vi "FPGA_main.vi"() -> ()   [LabVIEW 2019]
uses:
  trigger.ctl
  state.ctl
  <vilib>/rvi/Emulation/niFpgaGetClockAttributes.vi
  <vilib>/rvi/Emulation/niFpgaSctlEmulationGetInTimedLoop.vi
  <vilib>/rvi/Emulation/niFpgaEmulationReportErrorSimple.vi
  <vilib>/rvi/eio/common/nirviEmuTemplateMethod_errors.vi
  <vilib>/rvi/Emulation/niFpgaEmulationIsFPGAContextNoSignature.vi
  <vilib>/rvi/DataTransferAndStorage/Container/Common/niFpgaContainerGetUniqueNameForEmu.vi
  <vilib>/rvi/Memory/Memory_Emulation/niFpgaMemoryEmulationCacheClearOnFirstRun.vi
  <vilib>/rvi/Memory/Memory_Emulation/nirvimemoryEmulationManagerCache_MakeExclusive.vi
  <vilib>/rvi/Memory/Memory_Emulation/niFpgaMemoryEmulationValidateCache.vi
  <vilib>/rvi/Memory/Memory_Emulation/nirvimemoryEmulationManagerCache_InsertValue.vi
  <vilib>/Utility/error.llb/Clear Errors.vi
  <vilib>/rvi/Memory/Memory_Emulation/nirvimemoryEmulationManagerCache_ReleaseExclusive.vi
  <vilib>/rvi/Memory/Memory_Emulation/nirvimemoryEmulationManagerCache_GetValue.vi
  <vilib>/rvi/Memory/Memory_Emulation/nirvimemoryEmulationManagerCache_SetValue.vi
  <vilib>/rvi/Emulation/niFpgaProcessEmulError.vi
  <vilib>/rvi/Memory/Memory_Emulation/nirvimemoryFastEmulation.vi
  <vilib>/rvi/Memory/Memory_Emulation/nirvimemoryEmulation.vi
  <vilib>/rvi/errors/nirviReportUnexpectedCaseInternalError (U32).vi
  <vilib>/rvi/errors/niFpgaSetErrorForExecOnDevCompSimple.vi
  <vilib>/rvi/eio/common/nirviEmuReportErrorAndStop.vi
  <vilib>/rvi/FIFO/Fifo_Resource/nirvififoEmulationSetSize.vi
  <vilib>/rvi/FIFO/Fifo_Resource/nirviFifoEmulationQueueMgr.vi
  <instcachedir>/0/nirviFifoEmulationQueueMgr_E5CAEC123FF24DC58D834DCA3CDAA9B5.lvgen/nirviFifoEmulationQueueMgr_E5CAEC123FF24DC58D834DCA3CDAA9B5_002.vi
  <vilib>/rvi/FIFO/Fifo_Resource/nirvififoEmulationDetermineInputValidOut.vi
  <vilib>/rvi/FIFO/Fifo_Resource/nirvififoEmulationCreateLock.vi
  <vilib>/rvi/FIFO/Fifo_Resource/nirvififoEmulationObtainLock.vi
  <vilib>/rvi/FIFO/Fifo_Resource/nirvififoEmulationReleaseLock.vi
  <vilib>/rvi/occurrence/nirviWaitOnOccurrenceBase.vi
  <vilib>/rvi/errors/nirviReportUnexpectedCaseInternalError.vi
  <vilib>/rvi/Emulation/niFpgaCriticalErrorInLSC.vi
  <vilib>/rvi/interface/RandomDataEmulation/niFpgaRandomDataHandleErrors.vi
  <vilib>/eio/EIONode/EIONode.xnode
  <vilib>/rvi/DataTransferAndStorage/Container/XNode/niFpgaContainer.xnode
  <vilib>/rvi/DataTransferAndStorage/Register/Emulation/niFpgaRegisterEmulation.vi
  <vilib>/rvi/FIFO/Fifo_Resource/nirvififoEmulationWrite.vi
  <vilib>/rvi/FIFO/Fifo_Resource/nirvififoEmulationRead.vi
  <vilib>/rvi/interface/RandomDataEmulation/nirviRandomDataFpgaReadWriteTemplate.vi
panel:
  out "Numeric":u32
  in  "Samples":i16
  in  "Trigger":T1
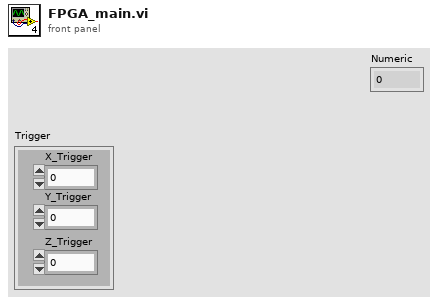
[diagram p1: front panel]
types:
  T1 = typedef "trigger.ctl" = cluster{"X_Trigger":i16, "Y_Trigger":i16, "Z_Trigger":i16}
  T2 = typedef "state.ctl" = enum16{"Send_fifo", "Send_memo", "Wait"}
  T3 = cluster{"X_Trigger":i16, "Y_Trigger":i16, "Z_Trigger":i16}
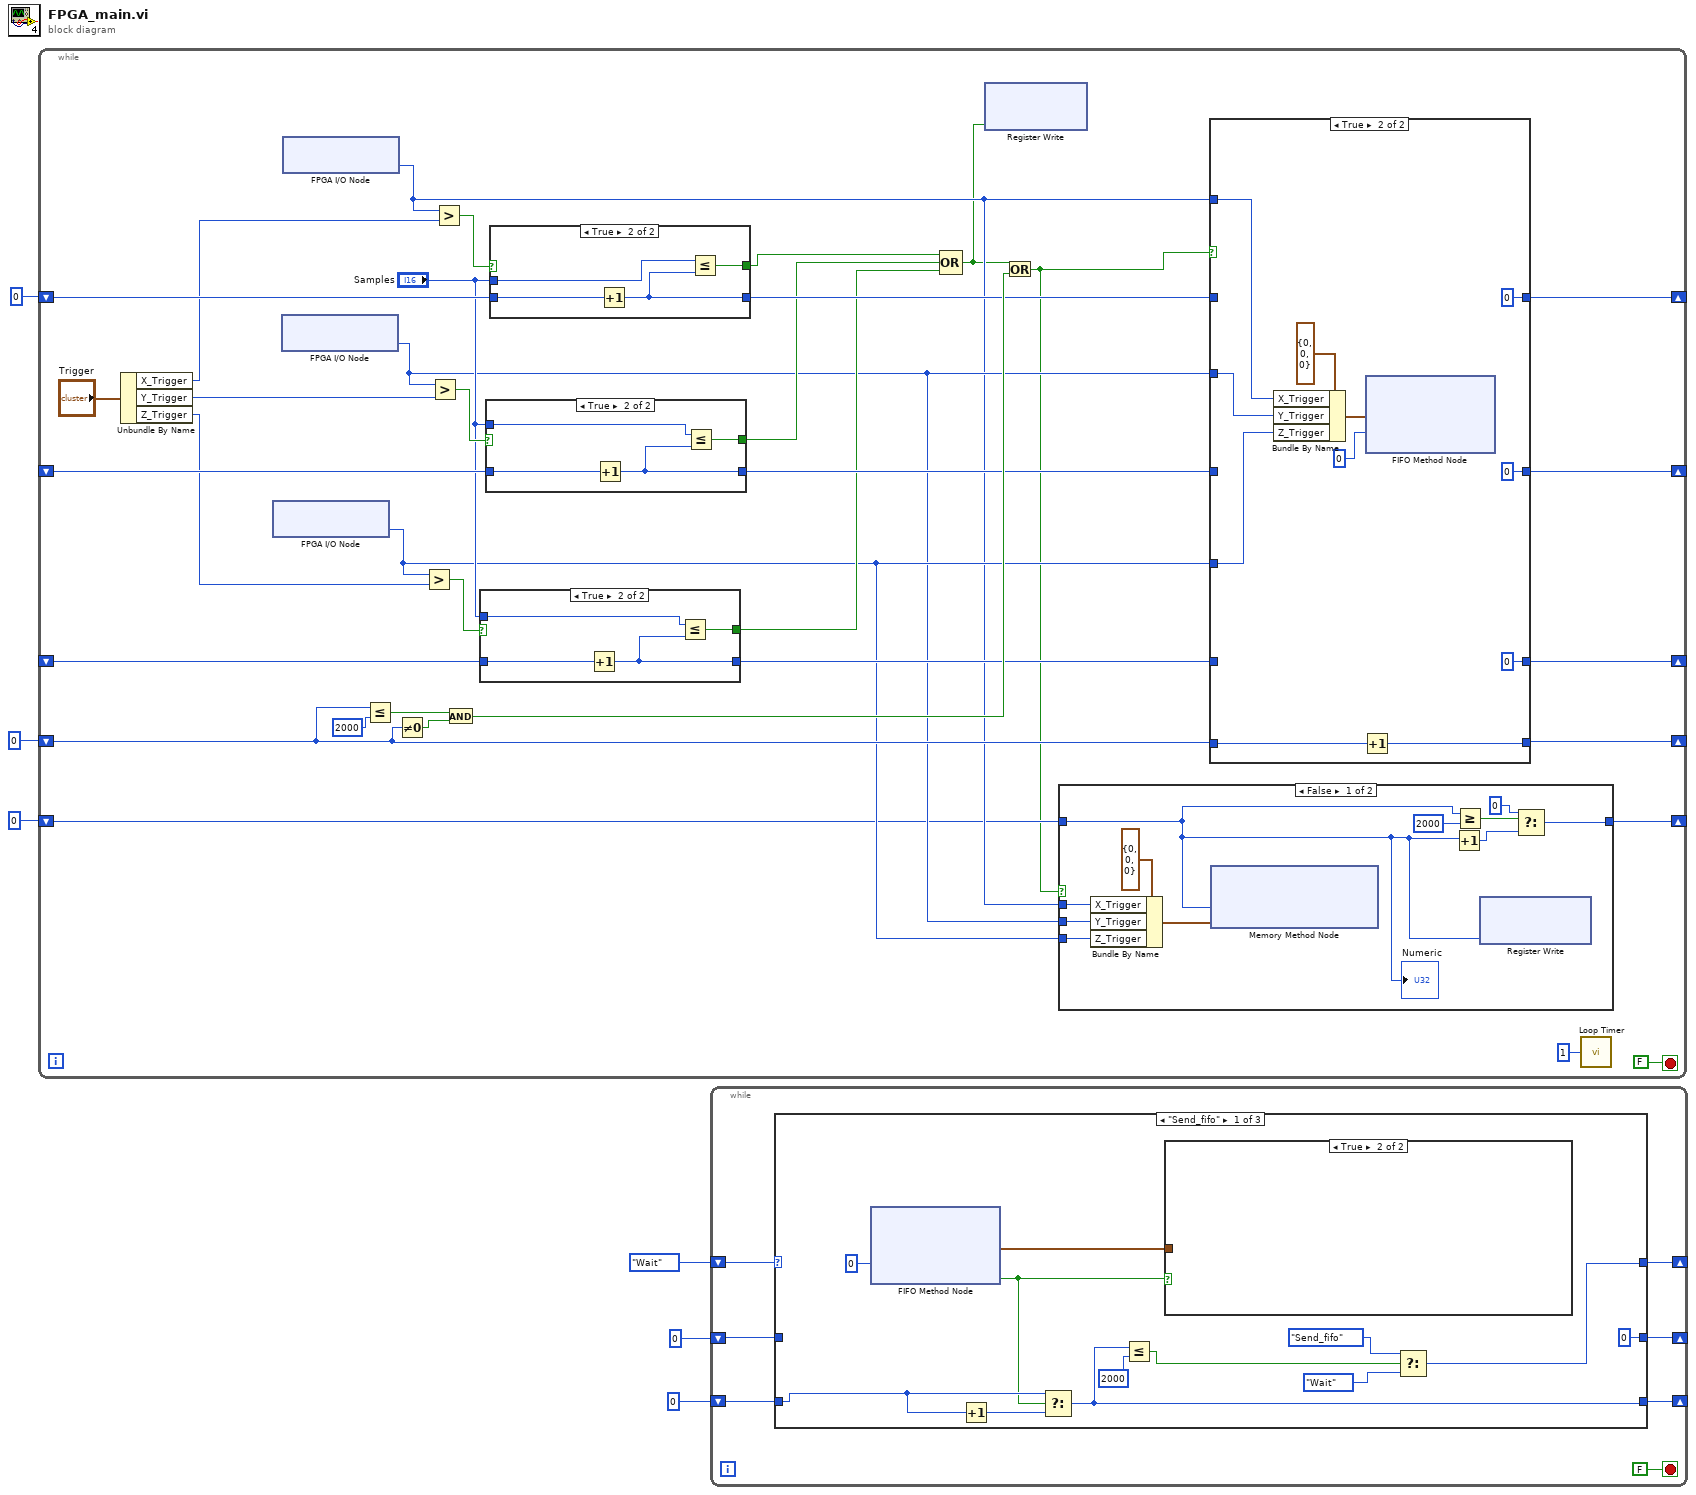
[diagram p0: block diagram]
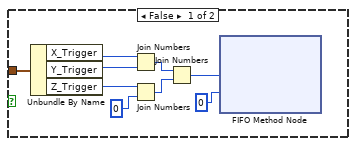
[diagram p2: hidden frame]
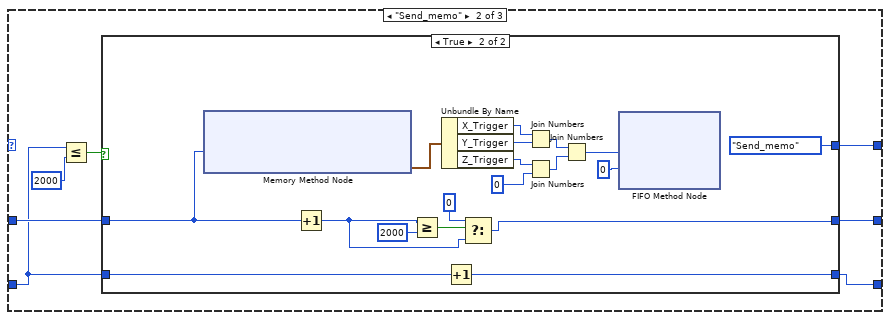
[diagram p3: hidden frame]
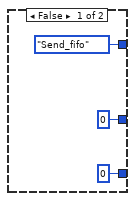
[diagram p4: hidden frame]
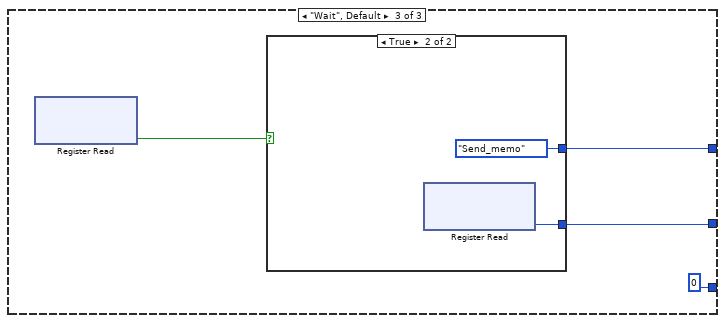
[diagram p5: hidden frame]
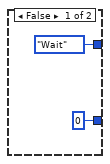
[diagram p6: hidden frame]
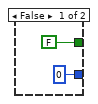
[diagram p8: hidden frame]
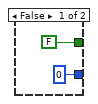
[diagram p9: hidden frame]
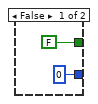
[diagram p10: hidden frame]
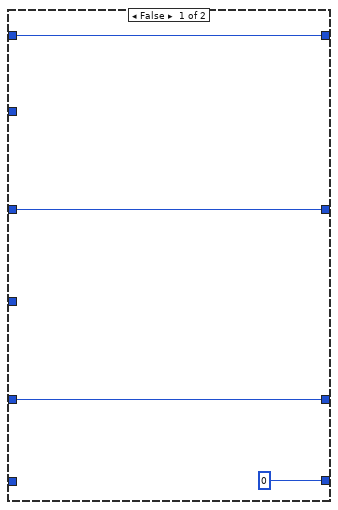
[diagram p11: hidden frame]
diagram:
  n1 = while {
    shift-right: [w41] -> _
    shift-left: i16 0 -> [w36]
    shift-right: [w31] -> _
    shift-left: i16 0 -> [w33]
    shift-right: [w26] -> _
    shift-left: _ -> [w28]
    shift-right: [w22] -> _
    shift-left: _ -> [w24]
    shift-right: [w9] -> _
    shift-left: u32 0 -> [w8]
    stop <- FALSE ("value") stop-if-true
    n2 = Unbundle By Name("Trigger") -> ("X_Trigger"=w18:i16, "Y_Trigger"=w17:i16, "Z_Trigger"=w16:i16)
    n3 = xnode "FPGA I/O Node"() -> ("AccelerationZ"=w13:i16)  [unwired: 1 in, 1 out]
    n4 = xnode "FPGA I/O Node"() -> ("AccelerationY"=w12:i16)  [unwired: 1 in, 1 out]
    n5 = xnode "FPGA I/O Node"() -> ("AccelerationX"=w11:i16)  [unwired: 1 in, 1 out]
    n6 = Less Or Equal?(x=w36, y=i16 2000) -> (x <= y?=w37:bool)
    n7 = Not Equal To 0?(x=w36) -> (x != 0?=w38:bool)
    n8 = Greater?(x=w13, y=w16) -> (0:w25:bool)
    n9 = Greater?(x=w12, y=w17) -> (0:w29:bool)
    n10 = Greater?(x=w11, y=w18) -> (0:w34:bool)
    n11 = And(x=w37, y=w38) -> (x .and. y?=w39:bool)
    n12 = case shown="True" w25 {
      tunnel: [FALSE w58] -> w19
      tunnel: w24 -> [_ w59]
      tunnel: [i16 0 w57] -> w23
      tunnel: "Samples" -> [_ w56]
      frame False {
      }
      frame True {
        n13 = Increment(x=w59) -> (x+1=w57:i16)
        n14 = Less Or Equal?(x=w56, y=w57) -> (x <= y?=w58:bool)
      }
    }
    n15 = case shown="True" w29 {
      tunnel: [FALSE w64] -> w20
      tunnel: w28 -> [_ w65]
      tunnel: [i16 0 w63] -> w27
      tunnel: "Samples" -> [_ w62]
      frame False {
      }
      frame True {
        n16 = Increment(x=w65) -> (x+1=w63:i16)
        n17 = Less Or Equal?(x=w62, y=w63) -> (x <= y?=w64:bool)
      }
    }
    n18 = case shown="True" w34 {
      tunnel: [FALSE w70] -> w21
      tunnel: w33 -> [_ w71]
      tunnel: [i16 0 w69] -> w32
      tunnel: "Samples" -> [_ w68]
      frame False {
      }
      frame True {
        n19 = Increment(x=w71) -> (x+1=w69:i16)
        n20 = Less Or Equal?(x=w68, y=w69) -> (x <= y?=w70:bool)
      }
    }
    n21 = Compound Arithmetic op=OR(w21, w20, w19) -> (w10:bool)
    n22 = xnode ("Register Write")("Data"=w10) -> ()  [unwired: 1 in, 1 out]
    n23 = Or(x=w10, y=w39) -> (x .or. y?=w7:bool)
    n24 = case shown="False" w7 {
      tunnel: w13 -> [w47 _]
      tunnel: w12 -> [w46 _]
      tunnel: w11 -> [w45 _]
      tunnel: [w44 w53] -> w9
      tunnel: w8 -> [w43 w53]
      frame False {
        n25 = Bundle By Name(cluster=T3 {"X_Trigger"=0, "Y_Trigger"=0, "Z_Trigger"=0} ("Data"), "X_Trigger"=w45, "Y_Trigger"=w46, "Z_Trigger"=w47) -> (w52:T3)
        n26 = xnode ("Memory Method Node")("Address"=w43, "Data"=w52) -> ()  [unwired: 1 in, 1 out]
        n27 = Increment(x=w43) -> (x+1=w42:u32)
        n28 = Greater Or Equal?(x=w43, y=u32 2000) -> (x >= y?=w49:bool)
        n29 = xnode ("Register Write")("Data"=w43) -> ()  [unwired: 1 in, 1 out]
        n30 = Select(t=u32 0, s=w49, f=w42) -> (s? t:f=w44:u32)
        "Numeric" <- w43
      }
      frame True {
      }
    }
    n31 = case shown="True" w7 {
      tunnel: w11 -> [_ w78]
      tunnel: w36 -> [_ w86]
      tunnel: [i16 0 w85] -> w41
      tunnel: [w74 i16 0] -> w31
      tunnel: w32 -> [w74 _]
      tunnel: [w73 i16 0] -> w26
      tunnel: w27 -> [w73 _]
      tunnel: w12 -> [_ w77]
      tunnel: [w72 i16 0] -> w22
      tunnel: w23 -> [w72 _]
      tunnel: w13 -> [_ w76]
      frame False {
      }
      frame True {
        n32 = Bundle By Name(cluster=T3 {"X_Trigger"=0, "Y_Trigger"=0, "Z_Trigger"=0} ("Element"), "X_Trigger"=w78, "Y_Trigger"=w77, "Z_Trigger"=w76) -> (w80:T3)
        n33 = Increment(x=w86) -> (x+1=w85:i16)
        n34 = xnode ("FIFO Method Node")("Element"=w80, "Timeout"=0) -> ()  [unwired: 1 in, 2 out]
      }
    }
    n35 = call "Loop Timer"("Count(mSec)"=u16 1) -> ()  [unwired: 1 out]
  }
  n36 = while {
    shift-right: [w91] -> _
    shift-left: state."Wait" ("State") -> [w92]
    shift-right: [w89] -> _
    shift-left: u32 0 ("Data") -> [w90]
    shift-right: [w87] -> _
    shift-left: u32 0 ("Data") -> [w88]
    stop <- FALSE stop-if-true
    n37 = case shown="\"Send_fifo\"" w92 {
      tunnel: [w94 w121 w145] -> w91
      tunnel: w90 -> [_ w120 _]
      tunnel: [u32 0 ("Data") w119 w143] -> w89
      tunnel: w88 -> [w102 w116 _]
      tunnel: [w100 w115 u32 0 ("Data")] -> w87
      frame "Send_fifo" {
        n38 = xnode ("FIFO Method Node")("Timeout"=0) -> ("Element"=w105:T3, "Timed Out?"=w98:bool)  [unwired: 1 in, 1 out]
        n39 = Increment(x=w102) -> (x+1=w101:u32)
        n40 = Select(t=w102, s=w98, f=w101) -> (s? t:f=w100:u32)
        n41 = Less Or Equal?(x=w100, y=u32 2000) -> (x <= y?=w97:bool)
        n42 = case shown="True" w98 {
          tunnel: w105 -> [w113 _]
          frame False {
            n43 = Unbundle By Name(w113) -> ("X_Trigger"=w112:i16, "Y_Trigger"=w111:i16, "Z_Trigger"=w110:i16)
            n44 = Join Numbers(hi=w112, lo=w111) -> ((hi.lo)=w107:u32)
            n45 = Join Numbers(hi=w110, lo=i16 0) -> ((hi.lo)=w106:u32)
            n46 = Join Numbers(hi=w107, lo=w106) -> ((hi.lo)=w108:u64)
            n47 = xnode ("FIFO Method Node")("Element"=w108, "Timeout"=0) -> ()  [unwired: 1 in, 2 out]
          }
          frame True {
          }
        }
        n48 = Select(t=state."Send_fifo" ("State"), s=w97, f=state."Wait") -> (s? t:f=w94:T2)
      }
      frame "Send_memo" {
        n49 = Less Or Equal?(x=w116, y=u32 2000) -> (x <= y?=w118:bool)
        n50 = case shown="True" w118 {
          tunnel: [state."Send_fifo" ("State") state."Send_memo" ("State")] -> w121
          tunnel: w120 -> [_ w132]
          tunnel: [u32 0 w127] -> w119
          tunnel: w116 -> [_ w126]
          tunnel: [u32 0 w125] -> w115
          frame False {
          }
          frame True {
            n51 = xnode ("Memory Method Node")("Address"=w132) -> ("Data"=w137:T3)  [unwired: 1 in, 1 out]
            n52 = Increment(x=w132) -> (x+1=w128:u32)
            n53 = Greater Or Equal?(x=w128, y=u32 2000) -> (x >= y?=w130:bool)
            n54 = Unbundle By Name(w137) -> ("X_Trigger"=w136:i16, "Y_Trigger"=w135:i16, "Z_Trigger"=w134:i16)
            n55 = Increment(x=w126) -> (x+1=w125:u32)
            n56 = Select(t=u32 0 ("y"), s=w130, f=w128) -> (s? t:f=w127:u32)
            n57 = Join Numbers(hi=w136, lo=w135) -> ((hi.lo)=w140:u32)
            n58 = Join Numbers(hi=w134, lo=i16 0) -> ((hi.lo)=w139:u32)
            n59 = Join Numbers(hi=w140, lo=w139) -> ((hi.lo)=w138:u64)
            n60 = xnode ("FIFO Method Node")("Element"=w138, "Timeout"=0) -> ()  [unwired: 1 in, 2 out]
          }
        }
      }
      frame "Wait", Default {
        n61 = xnode ("Register Read")() -> ("Data"=w146:bool)  [unwired: 1 in, 1 out]
        n62 = case shown="True" w146 {
          tunnel: [state."Wait" ("State") state."Send_memo" ("State")] -> w145
          tunnel: [u32 0 ("Data") w149] -> w143
          frame False {
          }
          frame True {
            n63 = xnode ("Register Read")() -> ("Data"=w149:u32)  [unwired: 1 in, 1 out]
          }
        }
      }
    }
  }
